vi "Upload.vi"(7 "Node-ID":u8, 10 "Multiplexer":cluster{"Index":u16, "Sub-Index":u8} {"Sub-Index" format="%.0x"; "Index" format="%.0x"}, 11 "Service Data Object in":refnum<class "Service Data Object.lvclass">) -> (1 "Request":refnum<class "CANopen Request Message.lvclass">, 2 "Expected Response":refnum<class "CANopen Response Message.lvclass">, 3 "Service Data Object out":refnum<class "Service Data Object.lvclass">)   [LabVIEW 2024, in "Service Data Object.lvclass"]
uses:
  Service Data Object.lvclass
  Service Data Object.lvclass/Service Data Object.ctl
  Initiate Down-Upload Response Comparator/Initiate Down-Upload Response Comparator.lvclass
  CANopen Request/CANopen Request Message.lvclass
  CANopen Message/CANopen Message.lvclass
  source/Typedefs/Function Code.ctl
  source/CANopen.lvlib
  SDO Response Compare Strategy/SDO Response Compare Strategy.lvclass
  CANopen Response/CANopen Response Message.lvclass
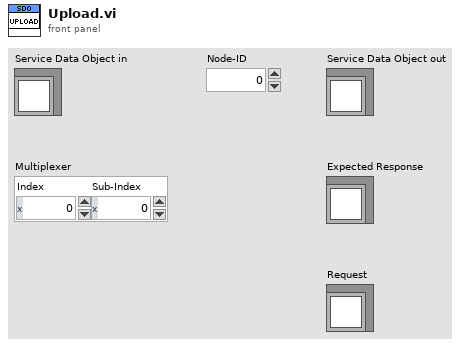
[diagram p1: front panel]
types:
  T1 = typedef "CANopen.lvlib/Function Code.ctl" = u8
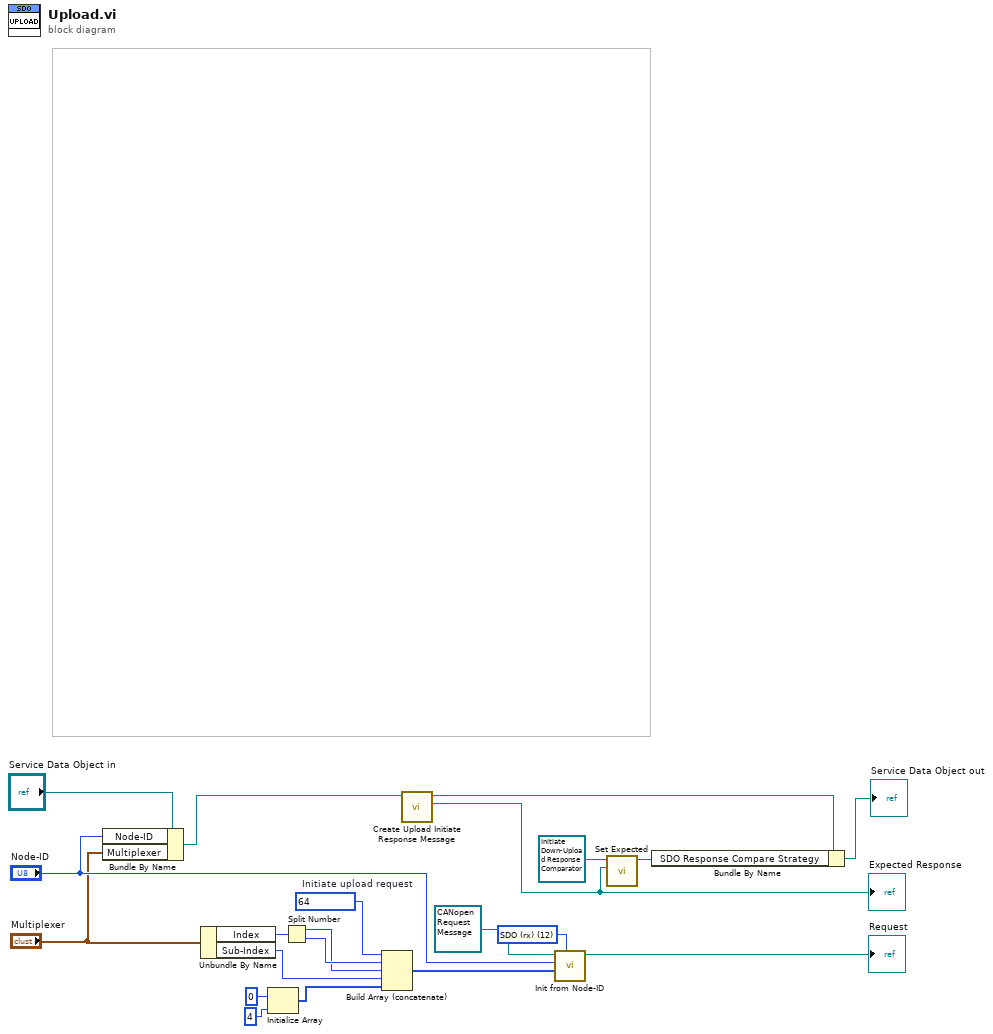
[diagram p0: block diagram]
diagram:
  w14 = T1 12 items=["NMT"=0, "EMCY/SYNC"=1, "TIME"=2, "PDO1 (tx)"=3, "PDO1 (rx)"=4, "PDO2 (tx)"=5, "PDO2 (rx)"=6, "PDO3 (tx)"=7, "PDO3 (rx)"=8, "PDO4 (tx)"=9, "PDO4 (rx)"=10, "SDO (tx)"=11, "SDO (rx)"=12, "NMT error control"=14] ("Function code")
  w12 = u8 64  # Initiate upload request
  n1 = Bundle By Name(cluster="Service Data Object in", "Node-ID"="Node-ID", "Multiplexer"="Multiplexer") -> (w8:refnum<class "Service Data Object.lvclass">)
  n2 = Unbundle By Name("Multiplexer") -> ("Index"=w21:u16, "Sub-Index"=w18:u8)
  n3 = Initialize Array(u8 0, 4 ("y")) -> (w16:u8[])
  n4 = Split Number(x=w21) -> (hi(x)=w19:u8, lo(x)=w20:u8)
  n5 = Build Array (concatenate)(w12, w20, w19, w18, w16) -> (w13:u8[])
  n6 = call "Create Upload Initiate Response Message.vi"("Service Data Object in"=w8) -> ("Response Message"=w2:refnum<class "CANopen Response Message.lvclass">, "Service Data Object out"=w4:refnum<class "Service Data Object.lvclass">)  [unwired: 9 in]
  "Expected Response" <- w2
  n7 = call "Init from Node-ID.vi"("Function Code"=w14, "Data"=w13, "Node-ID"="Node-ID", 11:refnum<class "CANopen Request Message.lvclass"> refnum ("CANopen Master.lvlib:CANopen Request Message.lvclass")) -> ("CANopen Message"=→"Request":refnum<class "CANopen Message.lvclass">)  [unwired: 7 in]
  n8 = call "Set Expected.vi"("CANopen Message"=w2, "SDO Response Compare Strategy in"=refnum<class "Initiate Down-Upload Response Comparator.lvclass"> refnum ("CANopen Master.lvlib:Initiate Down-Upload Response Comparator.lvclass")) -> ("SDO Response Compare Strategy out"=w5:refnum<class "Initiate Down-Upload Response Comparator.lvclass">)  [unwired: 9 in]
  n9 = Bundle By Name(cluster=w4, "SDO Response Compare Strategy"=w5) -> (→"Service Data Object out":refnum<class "Service Data Object.lvclass">)
